vi "XYposition_control1.4.vi"() -> ()   [LabVIEW 2014]
uses:
  <vilib>/Simulation/Scripting/Companion Diagram/SimConfigNode/SimParams.ctl
  <vilib>/Simulation/Scripting/Companion Diagram/SimConfigNode/_simSolvers.ctl
  <vilib>/Simulation/Implementation/Shared/SIMSCR Execution Mode.ctl
  <vilib>/Simulation/Param Hierarchy/Typedefs/SIMPH Param Control Actions.ctl
  <vilib>/Simulation/Implementation/Shared/SIM limit type.ctl
  <vilib>/myRIO/Common/Instrument Driver Framework/myRIO v1.0/Encoder/typedefs/Encoder Signal Mode.ctl
  <vilib>/myRIO/Instrument Drivers/Onboard IO/Encoder/typedefs/Encoder Reference.ctl
  <vilib>/myRIO/Common/Instrument Driver Framework/Utilities/typedefs/myRIO Generic Hardware Reference.ctl
  <vilib>/myRIO/Common/Instrument Driver Framework/Utilities/typedefs/Hardware Version Enum.ctl
  <vilib>/myRIO/Common/Instrument Driver Framework/Utilities/typedefs/myRIO v1.0 Reference.ctl
  <vilib>/myRIO/Common/Instrument Driver Framework/Utilities/typedefs/Generic FPGA Reference.ctl
  <vilib>/myRIO/Common/Instrument Driver Framework/myRIO v1.0/Encoder/typedefs/Encoder Channels Enum.ctl
  <vilib>/myRIO/Common/Instrument Driver Framework/myRIO v1.0/Encoder/typedefs/Encoder Configuration v1.0.ctl
  <vilib>/userdefined/High Color/nirio_resource_hc.ctl
  <vilib>/myRIO/Instrument Drivers/Onboard IO/PWM/typedefs/PWM Reference.ctl
  <vilib>/myRIO/Common/Instrument Driver Framework/myRIO v1.0/PWM/typedefs/PWM Channels Enum.ctl
  <vilib>/myRIO/Instrument Drivers/Onboard IO/PWM/typedefs/PWM Configuration.ctl
  <vilib>/myRIO/Instrument Drivers/Onboard IO/DIO/typedefs/DIO Reference.ctl
  <vilib>/myRIO/Common/Instrument Driver Framework/myRIO v1.0/DIO/typedefs/DIO Channels List.ctl
  <vilib>/myRIO/Common/Instrument Driver Framework/myRIO v1.0/DIO/typedefs/DIO Channels Enum.ctl
  <vilib>/Platform/TimedLoop/XDataNode/timing_clust.ctl
  <vilib>/Platform/TimedLoop/XDataNode/nitl_modes.ctl
  <vilib>/Platform/TimedLoop/XDataNode/wakeup.ctl
  <vilib>/Simulation/Implementation/Shared/NILVSim_ParamChanged.vi
  <vilib>/Simulation/Implementation/Shared/NILVSIM_BeginStep.vi
  <vilib>/myRIO/Common/Instrument Driver Framework/Utilities/vis/Is FPGA Ref Available.vi
  <vilib>/myRIO/Common/Instrument Driver Framework/myRIO v1.0/Encoder/vis/myRIO v1.1 Open Encoder.vi
  <vilib>/myRIO/Instrument Drivers/Onboard IO/Encoder/vis/Read.vi
  <vilib>/Simulation/Utility/Implementation/SIM Halt.vi
  <vilib>/Simulation/DataSources/Implementation/NILVSim Sine Wave.llb/SIM Sine Wave (scalar).vi
  <vilib>/Simulation/ContinuousLinear/Implementation/NILVSim Integrator new.llb/SIM Integrator distributor (scalar).vi
  <vilib>/Simulation/Implementation/Shared/SIM Is Init or Final Stage.vi
  <vilib>/Simulation/SignalArithmetic/Implementation/NILVSim Gain.llb/SIM Gain (scalar).vi
  <vilib>/Simulation/ContinuousLinear/Implementation/NILVSim Integrator new.llb/SIM Integrator collector (scalar).vi
  <vilib>/Simulation/ContinuousLinear/Implementation/NILVSim Derivative.llb/SIM derivative (scalar).vi
  <vilib>/myRIO/Common/Instrument Driver Framework/myRIO v1.0/DIO/vis/myRIO v1.1 Open DIO.vi
  <vilib>/myRIO/Instrument Drivers/Onboard IO/DIO/vis/Write.vi
  <vilib>/myRIO/Common/Instrument Driver Framework/myRIO v1.0/PWM/vis/myRIO v1.1 Open PWM.vi
  <vilib>/myRIO/Instrument Drivers/Onboard IO/PWM/vis/Set Duty Cycle and Frequency.vi
  <vilib>/Simulation/Implementation/Shared/NILVSim_Manager.vi
  <vilib>/Utility/error.llb/Clear Errors.vi
  <vilib>/Simulation/Implementation/Shared/NILVSim_FinalizeModel.vi
  <vilib>/Simulation/Implementation/Shared/NILVSim_FinishedLate.vi
  <vilib>/myRIO/Common/Instrument Driver Framework/Utilities/vis/Validate Channels.vi
  <vilib>/myRIO/Common/Instrument Driver Framework/myRIO v1.0/Encoder/vis/myRIO v1.0 Reserve Encoder.vi
  <vilib>/myRIO/Common/Instrument Driver Framework/myRIO v1.0/DIO/vis/myRIO v1.0 Reserve DIO.vi
  <vilib>/myRIO/Common/Instrument Driver Framework/myRIO v1.0/PWM/vis/myRIO v1.0 Reserve PWM.vi
  <vilib>/myRIO/Common/Instrument Driver Framework/myRIO v1.0/Encoder/vis/myRIO v1.0 Build MUX Configuration Encoder.vi
  <vilib>/myRIO/Common/Instrument Driver Framework/myRIO v1.0/Resource Manager/vis/myRIO v1.0 Reserve Channel List.vi
  <vilib>/myRIO/Common/Instrument Driver Framework/myRIO v1.0/DIO/vis/myRIO v1.0 Build MUX Configuration DIO.vi
  <vilib>/myRIO/Common/Instrument Driver Framework/myRIO v1.0/PWM/vis/myRIO v1.0 Build MUX Configuration PWM.vi
  <vilib>/myRIO/Common/Instrument Driver Framework/myRIO v1.0/Resource Manager/vis/myRIO v1.0 Create Configuration List.vi
  <vilib>/myRIO/Common/Instrument Driver Framework/myRIO v1.0/Resource Manager/vis/myRIO v1.0 Reserve Channel.vi
  <vilib>/myRIO/Common/Instrument Driver Framework/myRIO v1.0/Resource Manager/vis/myRIO v1.0 Unreserve Channel.vi
  <vilib>/myRIO/Common/Instrument Driver Framework/myRIO v1.0/Resource Manager/vis/myRIO v1.0 Build Mutex Name.vi
  <vilib>/Utility/file.llb/Read From Spreadsheet File (DBL).vi
  <vilib>/Simulation/Implementation/Shared/SIM Unbundle Sim Info.vi
  <vilib>/Simulation/Implementation/Shared/SIMSH Read Queue.vi
  <vilib>/Simulation/Implementation/Shared/NILVSim_Initialize.vi
  <vilib>/Utility/VariantDataType/GetNumericInfo.vi
  <vilib>/Utility/error.llb/Error Cluster From Error Code.vi
  <vilib>/myRIO/Common/Instrument Driver Framework/myRIO v1.0/myRIO v1.1 Open.vi
  <vilib>/myRIO/Common/Instrument Driver Framework/Utilities/vis/IO Manager.vi
  <vilib>/myRIO/Common/Instrument Driver Framework/Utilities/vis/Configuration Manager.vi
  <vilib>/myRIO/Common/Instrument Driver Framework/myRIO v1.0/Resource Manager/vis/myRIO v1.0 Configure IO.vi
  <vilib>/myRIO/Common/Instrument Driver Framework/myRIO v1.0/myRIO v1.0 Close.vi
  <vilib>/myRIO/Common/Instrument Driver Framework/myRIO v1.0/Encoder/vis/myRIO v1.0 Configure Encoder.vi
  <vilib>/myRIO/Common/Instrument Driver Framework/myRIO v1.0/Encoder/vis/myRIO v1.0 Read Encoder.vi
  <vilib>/Simulation/Utility/Implementation/NILVSim Get Time and IsAcceptedStep.vi
  <vilib>/myRIO/Common/Instrument Driver Framework/myRIO v1.0/DIO/vis/myRIO v1.0 Write DIO.vi
  <vilib>/myRIO/Common/Instrument Driver Framework/myRIO v1.0/PWM/vis/myRIO v1.0 Write PWM.vi
  <vilib>/Simulation/Implementation/Shared/NILVSim_GetModelError.vi
  <vilib>/Simulation/Implementation/Shared/SIM Bundle Sim Info.vi
  <vilib>/Simulation/Scripting/Companion Diagram/SimConfigNode/SimDog.xnode
  <vilib>/Platform/TimedLoop/XDataNode/XDataNode.xnode
  <vilib>/myRIO/Express VI/Onboard IO/Encoder/Encoder Express VI.xnode
  <vilib>/myRIO/Instrument Drivers/Onboard IO/Encoder/vis/myRIO Encoder Open.xnode
  <vilib>/myRIO/Common/Instrument Driver Framework/myRIO v1.0/Encoder/typedefs/Encoder Count Direction Enum.ctl
  <vilib>/Simulation/Implementation/XNodeFramework/SimXNode/SimX.xnode
  <vilib>/myRIO/Express VI/Onboard IO/DO/DO Express VI.xnode
  <vilib>/myRIO/Instrument Drivers/Onboard IO/DIO/vis/myRIO DIO Open.xnode
  <vilib>/myRIO/Express VI/Onboard IO/PWM/PWM Express VI.xnode
  <vilib>/myRIO/Instrument Drivers/Onboard IO/PWM/vis/myRIO PWM Open.xnode
  <vilib>/myRIO/Instrument Drivers/Onboard IO/PWM/PWM.lvlib
  <vilib>/myRIO/Instrument Drivers/Onboard IO/DIO/DIO.lvlib
  <vilib>/Simulation/ContinuousLinear/Implementation/NILVSim Integrator new.llb/SIM Integrator (scalar).vi
  <vilib>/myRIO/Instrument Drivers/Onboard IO/Encoder/Encoder.lvlib
  <vilib>/Platform/TimedLoop/XDataNode/XDNodeRunTimeDep.lvlib
  <vilib>/Simulation/Implementation/Shared/NI_SIM_Implementation.lvlib
panel:
  in  "C - Count by this number":i32=30
  out "Duty Cycle 1":dbl
  out "LoopNumber":dbl
  in  "Pause":bool
  in  "Global stop":bool
  in  "VCA1gain":dbl=-10.0 format="%#_13g"
  out "Position load rate":dbl
  in  "VCA2gain":dbl=-10.0 format="%#_13g"
  in  "millisecond multiple":u32=2
  out "ArrayIndex":i32
  in  "Zero encoder 3":bool
  in  "VCA 1 DesiredPosition (um)":dbl
  in  "offset (um)":dbl format="%#_13g"
  in  "Position control or sinusoid 1":bool
  in  "frequency 3":dbl=3.0 format="%#_13g"
  in  "amplitude (um)":dbl=2000.0
  in  "PWM Frequency [Hz]":dbl=20000.0 format="%#_13g"
  in  "Zero encoder 2":bool
  in  "VCA 1 control on/off":bool
  out "Position (um)":dbl(slide) scale=-15000.0..15000.0
  in  "Ki 1":dbl
  out "Position (um) 2":dbl(graph)
  out "ActualPosition (um)":i32
  in  "Kd 1":dbl=3e-07 format="%#_13g"
  in  "Kp 1":dbl=0.00015
  in  "offset (um)":dbl format="%#_13g"
  in  "Position control or sinusoid 2":bool
  in  "frequency (Hz)":dbl=15.0 format="%#_13g"
  in  "amplitude (um)":dbl=100.0
  out "Position (um)2 2":dbl(slide) scale=-15000.0..15000.0
  in  "VCA2 control on/off":bool
  in  "Ki 2":dbl
  out "Position (um)2":dbl(graph)
  out "ActualPosition (um) 2":i32
  in  "Kd 2":dbl=3e-07 format="%#_13g"
  out "Duty Cycle 2":dbl
  in  "PWM Frequency [Hz] 2":dbl=20000.0 format="%#_13g"
  in  "VCA 2 desired position (um)":dbl
  in  "Kp 2":dbl=0.00015
  # "VCA 1 (bottom)"
  # "VCA 2 (top)"
  # "Sinusoid"
  # "Pos control"
  # "Pos control"
  # "Sinusoid"
  # "ON"
  # "OFF"
  # "OFF"
  # "ON"
  # "Pause"
  # "Unpause"
  # "Higher C makes it go faster"
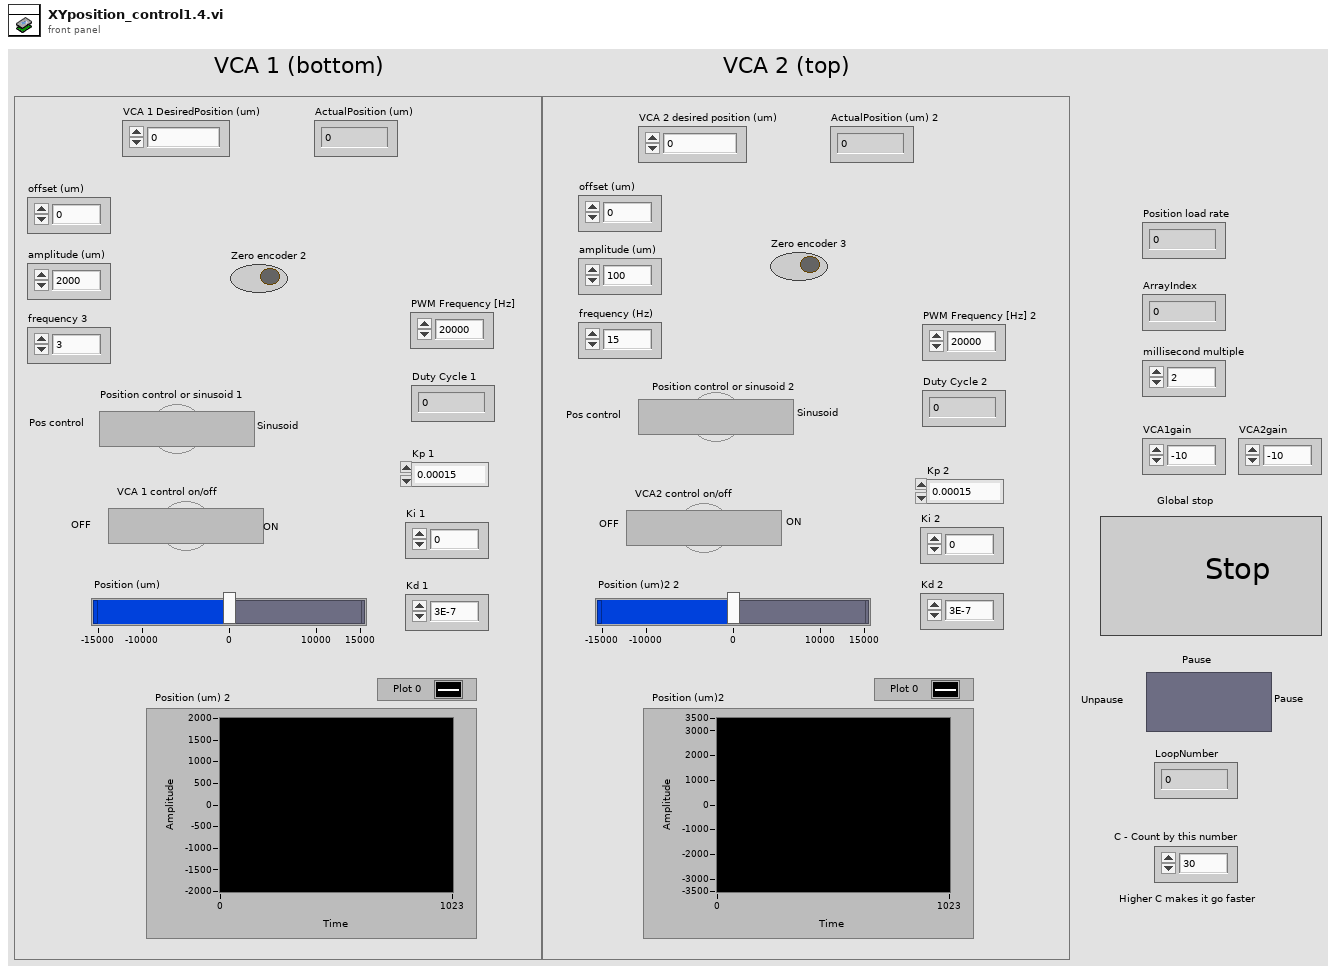
[diagram p1: front panel]
types:
  T1 = typedef "PWM.lvlib/PWM Reference.ctl" = cluster{"myRIO Reference":T2, "PWM Channels Enum":T6, "PWM Configuration":T7}
  T2 = typedef "myRIO Generic Hardware Reference.ctl" = cluster{"myRIO Model":T3, "myRIO Hardware Reference":T4}
  T3 = typedef "Hardware Version Enum.ctl" = enum16{"Unknown", "myRIO-1900", "myRIO-1950"}
  T4 = typedef "myRIO v1.0 Reference.ctl" = cluster{"Generic FPGA Reference":T5, "Allow multiple opens":bool}
  T5 = typedef "Generic FPGA Reference.ctl" = refnum<k20>
  T6 = typedef "PWM Channels Enum.ctl" = enum16{"Not Connected", "C/PWM0", "C/PWM1", "A/PWM0", "A/PWM1", "A/PWM2", "B/PWM0", "B/PWM1", "B/PWM2"}
  T7 = typedef "PWM.lvlib/PWM Configuration.ctl" = cluster{"Frequency":dbl, "Duty Cycle":dbl}
  T8 = typedef "nirio_resource_hc.ctl" = tag
  T9 = typedef "DIO.lvlib/DIO Reference.ctl" = cluster{"myRIO Reference":T2, "DIO Channels List":T10}
  T10 = typedef "DIO Channels List.ctl" = T11[]
  T11 = typedef "DIO Channels Enum.ctl" = enum16{"Not Connected", "C/DIO0", "C/DIO1", "C/DIO2", "C/DIO3", "C/DIO4", "C/DIO5", "C/DIO6", "C/DIO7", "A/DIO0", "A/DIO1", "A/DIO2", "A/DIO3", "A/DIO4", "A/DIO5", "A/DIO6", "A/DIO7", "A/DIO8", "A/DIO9", "A/DIO10", "A/DIO11", "A/DIO12", "A/DIO13", "A/DIO14", "A/DIO15", "B/DIO0", "B/DIO1", "B/DIO2", "B/DIO3", "B/DIO4", "B/DIO5", "B/DIO6", "B/DIO7", "B/DIO8", "B/DIO9", "B/DIO10", "B/DIO11", "B/DIO12", "B/DIO13", "B/DIO14", "B/DIO15", "LED0", "LED1", "LED2", "LED3", "Button0"}
  T12 = typedef "Encoder.lvlib/Encoder Reference.ctl" = cluster{"myRIO Reference":T2, "Encoder Channels Enum":T13}
  T13 = typedef "Encoder Channels Enum.ctl" = enum16{"Not Connected", "C/ENC0", "C/ENC1", "A/ENC", "B/ENC"}
  T14 = typedef "Encoder Signal Mode.ctl" = enum16{"Quadrature phase signal", "Step and direction signal"}
  T15 = typedef "SIMSCR Execution Mode.ctl" = enum16{"Simulate to Completion", "Single Time-Step Simulation (Fixed Step Only)"}
  T16 = typedef "SIMPH Param Control Actions.ctl" = enum16{"get params", "set params"}
  T17 = typedef "SIM limit type.ctl" = enum16{"upper", "lower", "both", "none"}
  T18 = typedef "SimParams.ctl" = cluster{"Initial Time (s)":dbl, "Final Time (s)":dbl, "Step Size (s)":dbl, "ODE Solver":T19, "Minimum Step Size (s)":dbl, "Maximum Step Size (s)":dbl, "Relative Tolerance":dbl, "Absolute Tolerance":dbl, "Software Timing":bool, "Initial Step Size (s)":dbl, "Automatic Fixed Step Size?":bool, "Automatic Discrete Step Size?":bool, "Discrete Step Size (s)":dbl, "Calculate using Time Step":bool, "Solver Wired?":bool, "Prev.Frm.Expected End":u64, "Prev.Frm.Actual End":u64, "Prev.Frm.Finished Late?":bool, "Prev.Iter.Expected End":u64, "Prev.Iter.Actual End":u64, "Prev.Iter.Finished Late?":bool, "Expected Iteration Start":u64, "Actual Iteration Start":u64, "Expected Frame Start":u64, "Actual Frame Start":u64, "Source Name":string, "Name":string, "Period":i64, "Deadline":i64, "Offset":i64, "Start":i64, "Priority":i32, "Timeout":i32, "Processor":i32, "Mode":enum32{"No Change", "Process missed periods, maintain original phase", "Discard missed periods, maintain original phase", "Process missed periods, ignore original phase", "Discard missed periods, ignore original phase"}, "Wakeup reason":enum32{"Normal", "Aborted", "Asynchronous wakeup", "Timing source error", "Timed loop error", "Timeout"}, "Error":errorcluster, "Source Type":string, "Secondary Source Type":string, "Global End Time":u64, "Global Start Time":u64, "Full Solver Reset":bool, "Execution Mode":T15, "Nan/Inf Check":bool, "Custom Solver Library":string, "Solver Is Variable":bool, "custom solver name":string, "Signal Collection Decimation":u32}
  T19 = typedef "_simSolvers.ctl" = enum16{"Runge-Kutta 1 (Euler)", "Runge-Kutta 2", "Runge-Kutta 3", "Runge-Kutta 4", "Runge-Kutta 23 (variable)", "Runge-Kutta 45 (variable)", "BDF (variable)", "Adams-Moulton (variable)", "Rosenbrock (variable)", "Discrete States Only", "SDIRK 4 (variable)", "Radau 5 (variable)", "Radau 9 (variable)", "Radau 13 (variable)", "Radau [Variable Order] (variable)", "Gear's Method (variable)", "Linearizer", "State Query", "Trim Eval", "Custom Solver"}
  T20 = typedef "XDNodeRunTimeDep.lvlib/timing_clust.ctl" = cluster{"Expected End [f-1]":u64, "Actual End [f-1]":u64, "Finished Late? [f-1]":bool, "Expected End [i-1]":u64, "Actual End [i-1]":u64, "Finished Late? [i-1]":bool, "Expected Start [i]":u64, "Actual Start [i]":u64, "Expected Start [f]":u64, "Actual Start [f]":u64, "Source Name":string, "Structure Name":string, "Period":i64, "Deadline":i64, "Offset":i64, "Start":i64, "Priority":i32, "Timeout":i32, "Mode":T21, "Wakeup Reason":T22, "Error":errorcluster, "Source Type":string, "Secondary Source Type":string, "Global End Time":u64, "Global Start Time":u64, "Frame Duration":u64, "Iteration Duration":u64, "Assigned CPU":i32, "I/O Scan Engine Mode":u32}
  T21 = typedef "XDNodeRunTimeDep.lvlib/nitl_modes.ctl" = enum32{"No Change", "Process missed periods, maintain original phase", "Discard missed periods, maintain original phase", "Process missed periods, ignore original phase", "Discard missed periods, ignore original phase"}
  T22 = typedef "XDNodeRunTimeDep.lvlib/wakeup.ctl" = enum32{"Normal", "Aborted", "Asynchronous wakeup", "Timing source error", "Timed loop error", "Timeout"}
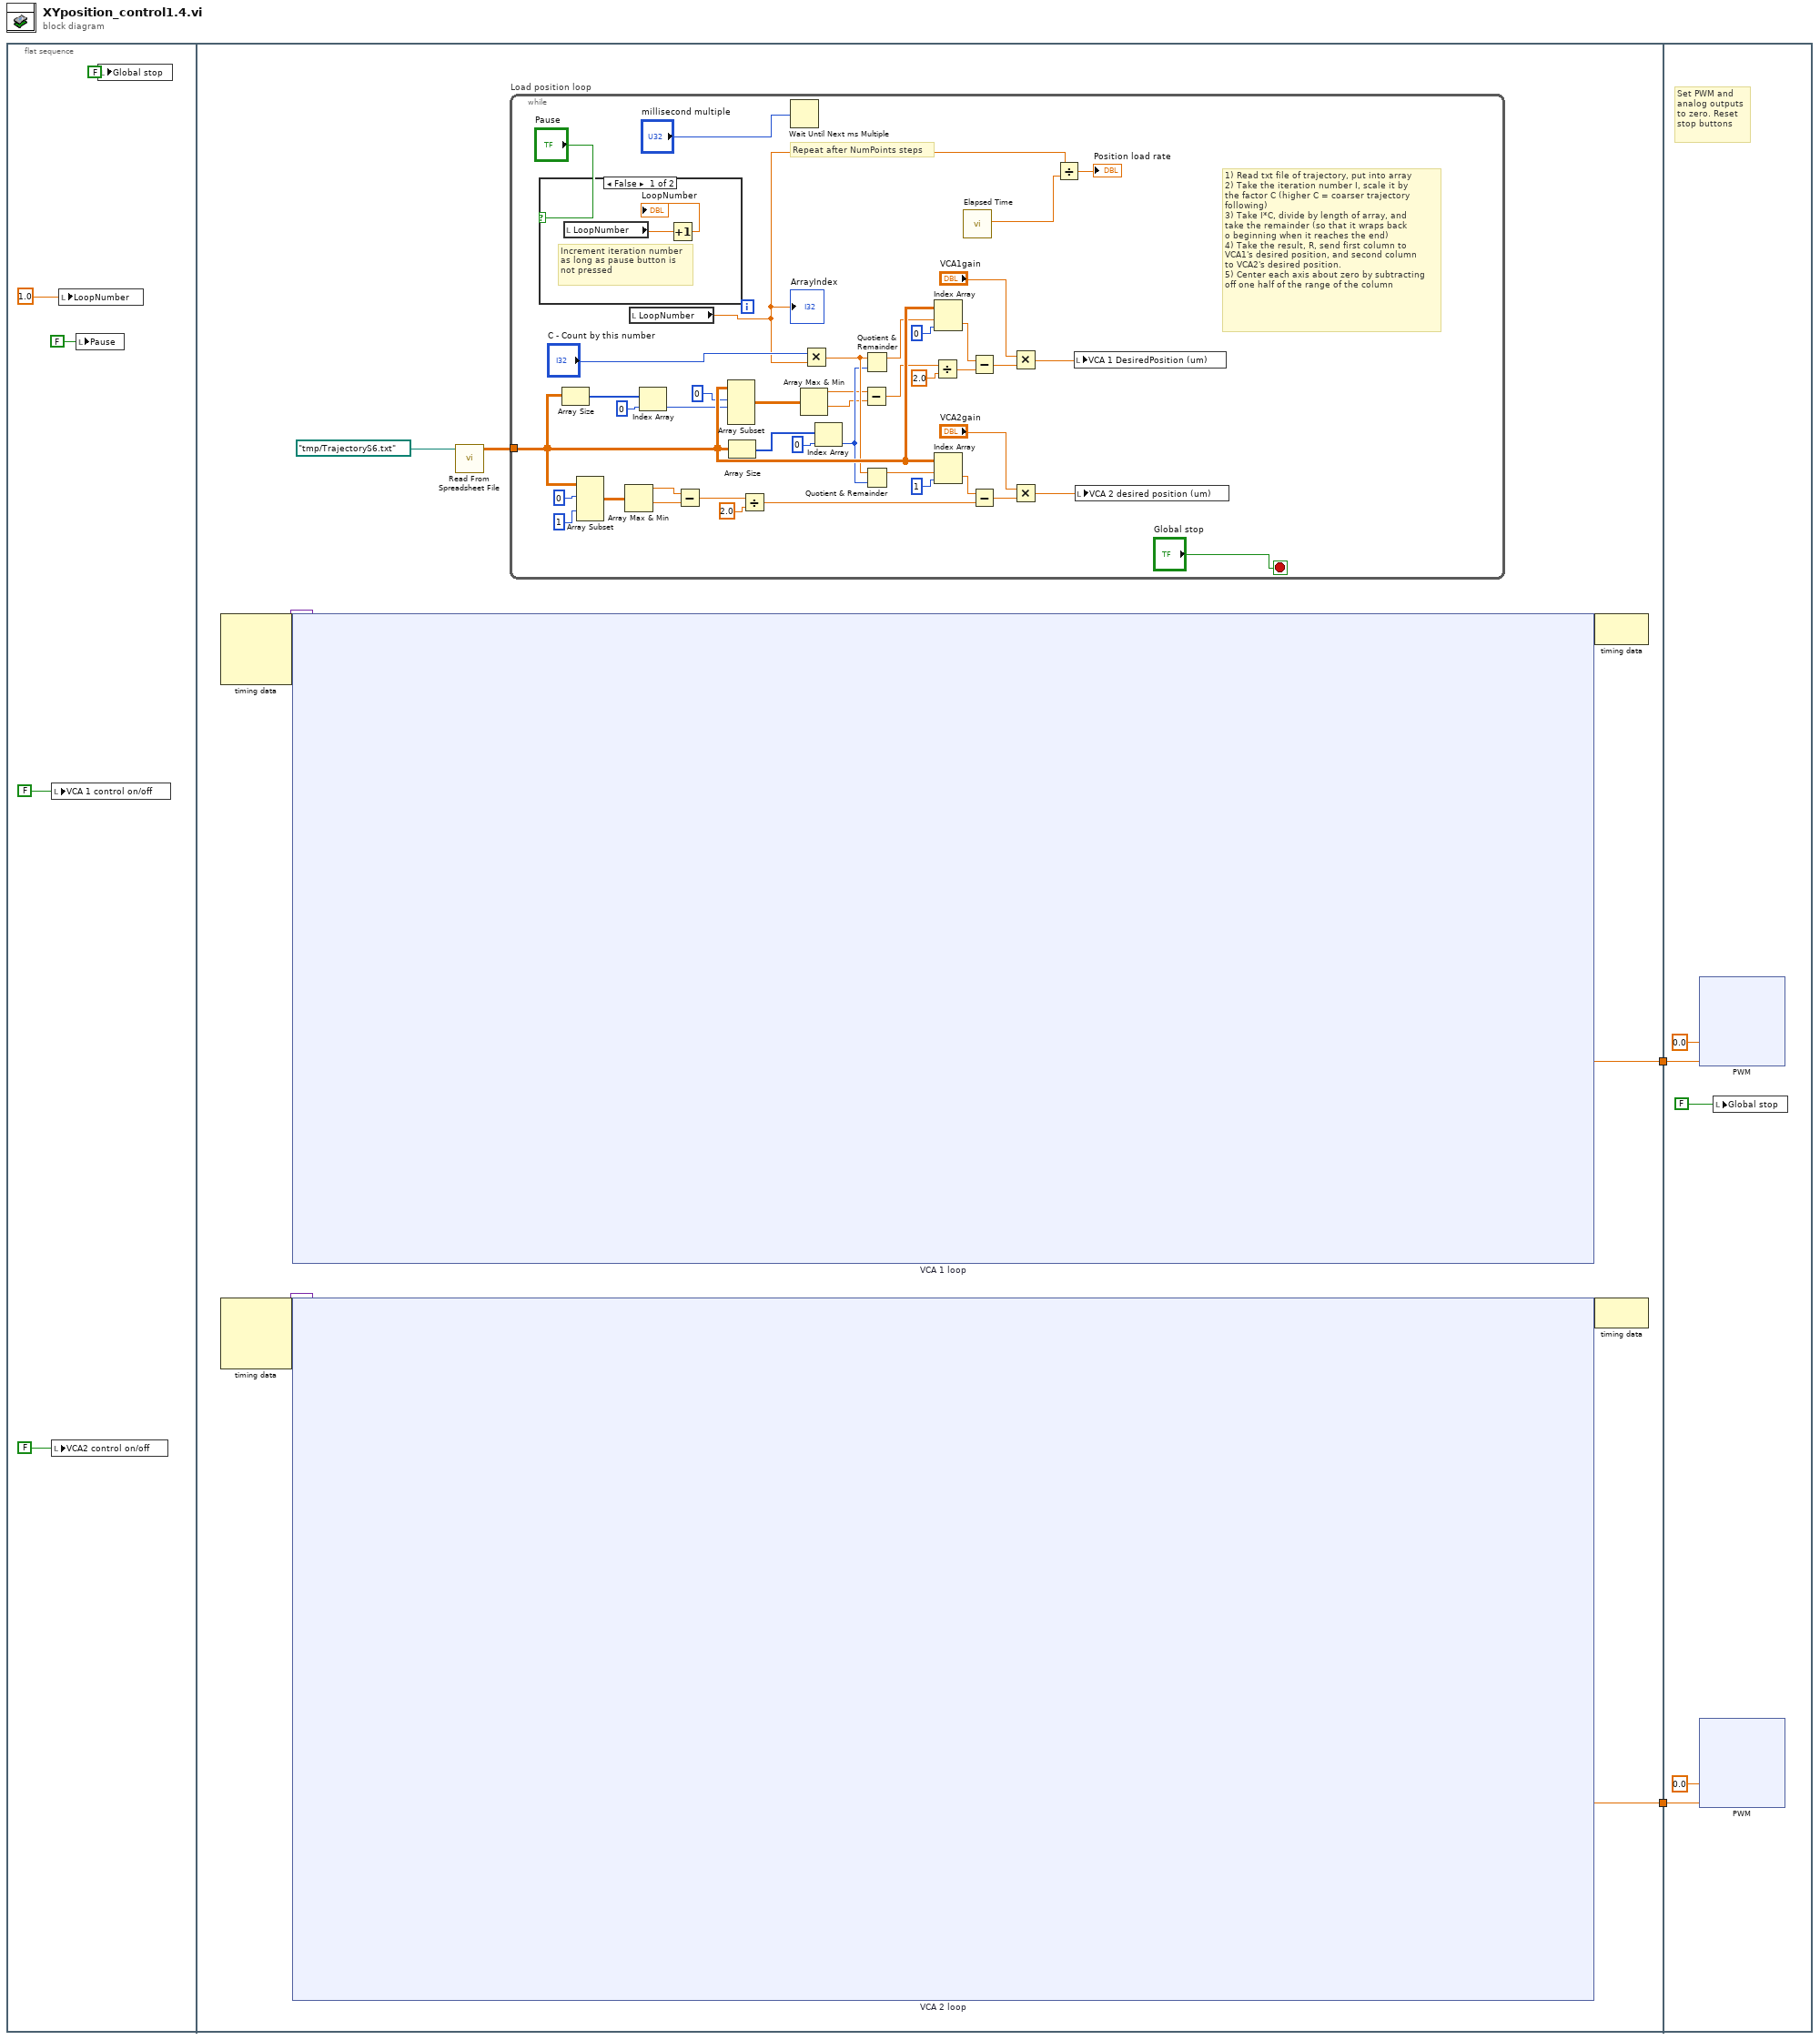
[diagram p0: block diagram]
diagram:
  n1 = flat-sequence {
    tunnel: [w13] -> w2
    tunnel: [w10] -> w1
    tunnel: w2 -> [w1995]
    tunnel: w1 -> [w1992]
    frame #0 {
      n2 = local write "VCA 1 control on/off"(FALSE ("VCA 1 control on/off")) -> ()
      n3 = local write "VCA2 control on/off"(FALSE ("VCA2 control on/off")) -> ()
      n4 = local write "LoopNumber"(1.0 ("LoopNumber")) -> ()
      n5 = local write "Pause"(FALSE ("Pause")) -> ()
      n6 = local write "Global stop"(FALSE ("Stop")) -> ()
    }
    frame #1 {
      n7 = node-c288() -> (w12:variant)  [unwired: 4 in]
      n8 = node-c288() -> (w15:variant)  [unwired: 4 in]
      n9 = node-c254 "VCA 1 loop"(w12) -> (w11:variant, w10:dbl)
      n10 = node-c254 "VCA 2 loop"(w15) -> (w14:variant, w13:dbl)
      n11 = call-poly <vilib>:"Read From Spreadsheet File.vi"("file path (dialog if empty)"=path "/tmp/TrajectoryS6.txt") -> ("all rows"=w8:dbl[][])  [unwired: 6 in, 4 out]
      n12 = while "Load position loop" {
        tunnel: w8 -> [w55]
        stop <- "Global stop" stop-if-true
        # "1) Read txt file of trajectory, put into array\n2) Take the iteration number I, scale it by \nthe factor C (higher C = coarser trajectory\nfollowing)\n3) Take I*C, divide by length of array, and \ntake the remainder (so that it wraps back \no beginning when it reaches the end)\n4) Take the result, R, send first column to \nVCA1's desired position, and second column \nto VCA2's desired position.\n5) Center each axis about zero by subtracting \noff one half of the range of the column"
        # "Repeat after NumPoints steps"
        n13 = case shown="False" "Pause" {
          frame False {
            # "Increment iteration number\nas long as pause button is\nnot pressed"
            n14 = local read "LoopNumber"() -> (w58:dbl)
            n15 = Increment(x=w58) -> (x+1=→"LoopNumber":dbl)
          }
          frame True {
            # "If Pause button is pressed,\npause incrementing iteration\nnumber"
          }
        }
        n16 = Array Size(array=w55) -> (size(s)=w35:i32[])
        n17 = Array Subset(array=w55, index (row)=0 ("index"), index (col)=1 ("index")) -> (w28:dbl[][])  [unwired: 2 in]
        n18 = Array Max & Min(array=w28) -> (max value=w27:dbl, min value=w26:dbl)  [unwired: 2 out]
        n19 = local read "LoopNumber"() -> (w16:dbl)
        "ArrayIndex" <- w16
        n20 = Index Array(array=w35, index=0) -> (element=w32:i32)
        n21 = Subtract(x=w27, y=w26) -> (x-y=w22:dbl)
        n22 = Array Subset(array=w55, index (row)=0 ("index"), length (row)=w32) -> (w29:dbl[][])  [unwired: 2 in]
        n23 = Array Size(array=w55) -> (size(s)=w37:i32[])
        n24 = Divide(x=w22, y=2.0) -> (x/y=w19:dbl)
        n25 = Wait Until Next ms Multiple(millisecond multiple="millisecond multiple") -> ()  [unwired: 1 out]
        n26 = Array Max & Min(array=w29) -> (max value=w25:dbl, min value=w24:dbl)  [unwired: 2 out]
        n27 = Multiply(x="C - Count by this number", y=w16) -> (x*y=w49:dbl)
        n28 = Index Array(array=w37, index=0) -> (element=w36:i32)
        n29 = Subtract(x=w25, y=w24) -> (x-y=w23:dbl)
        n30 = Quotient & Remainder(x=w49, y=w36) -> (x-y*floor(x/y)=w43:dbl)  [unwired: 1 out]
        n31 = Quotient & Remainder(x=w49, y=w36) -> (x-y*floor(x/y)=w47:dbl)  [unwired: 1 out]
        n32 = Divide(x=w23, y=2.0) -> (x/y=w21:dbl)
        n33 = Index Array(array=w55, index (row)=w43, index (col)=0 ("disabled index (col)")) -> (element=w50:dbl)
        n34 = Index Array(array=w55, index (row)=w47, index (col)=1 ("disabled index (col)")) -> (element=w53:dbl)
        n35 = call "Elapsed Time"() -> ("Elapsed Time (s)"=w41:dbl)  [unwired: 12 in, 7 out]
        n36 = Subtract(x=w50, y=w21) -> (x-y=w51:dbl)
        n37 = Subtract(x=w53, y=w19) -> (x-y=w54:dbl)
        n38 = Multiply(x="VCA1gain", y=w51) -> (x*y=w52:dbl)
        n39 = Multiply(x="VCA2gain", y=w54) -> (x*y=w48:dbl)
        n40 = Divide(x=w16, y=w41) -> (x/y=→"Position load rate":dbl)
        n41 = local write "VCA 1 DesiredPosition (um)"(w52) -> ()
        n42 = local write "VCA 2 desired position (um)"(w48) -> ()
      }
      n43 = node-c288(w11) -> ()  [unwired: 1 out]
      n44 = node-c288(w14) -> ()  [unwired: 1 out]
    }
    frame #2 {
      # "Set PWM and \nanalog outputs\nto zero. Reset \nstop buttons"
      n45 = xnode ("PWM")("Duty Cycle"=0.0, "Frequency [Hz]"=w1992) -> ()  [unwired: 1 in, 1 out]
      n46 = xnode ("PWM")("Duty Cycle"=0.0, "Frequency [Hz]"=w1995) -> ()  [unwired: 1 in, 1 out]
      n47 = local write "Global stop"(FALSE ("Stop")) -> ()
    }
  }
